vi "DateTimeMeasure.vi"(5 "EndTime":timestamp, 7 "StartTime":timestamp, 8 "error in":errorcluster, 11 "DateTimeMeasure":refnum<class "DateTimeMeasure.lvclass">) -> (0 "error out":errorcluster, 3 "Passed":bool)   [LabVIEW 2020]
uses:
  ProligentResultProcessor/Measure/DateTimeMeasure/DateTimeMeasure.lvclass
  C:/Projects/Result Processor/src/LabVIEWResultProcessor/ProligentResultProcessor/Measure/Measure/Measure.lvclass
  ProligentResultProcessor/Measure/DateTimeMeasureLimit/DateTimeMeasureLimit.lvclass
  C:/Projects/Result Processor/src/LabVIEWResultProcessor/ProligentResultProcessor/Measure/RangeMeasureLimit/RangeMeasureLimit.lvclass
  C:/Projects/Result Processor/src/LabVIEWResultProcessor/ProligentResultProcessor/Measure/MeasureLimit/MeasureLimit.lvclass
  ProligentResultProcessor/Measure/RangeMeasureLimit/ComparisonType.ctl
  ProligentResultProcessor/Measure/Measure/SetStartDate.vi
  ProligentResultProcessor/Measure/Measure/SetMeasureExecutionStatus.vi
  ProligentResultProcessor/Measure/DateTimeMeasure/SetValue.vi
  ProligentResultProcessor/Measure/Measure/SetComments.vi
  ProligentResultProcessor/Measure/Measure/SetMeasureId.vi
  ProligentResultProcessor/Measure/Measure/GetStartDate.vi
  ProligentResultProcessor/Measure/Measure/GetMeasureExecutionStatus.vi
  ProligentResultProcessor/Measure/DateTimeMeasure/GetValue.vi
  ProligentResultProcessor/Measure/Measure/GetComments.vi
  ProligentResultProcessor/Measure/Measure/GetMeasureId.vi
  ProligentResultProcessor/Measure/Measure/GetLimit.vi
  ProligentResultProcessor/Measure/DateTimeMeasureLimit/SetHigherBound.vi
  ProligentResultProcessor/Measure/DateTimeMeasureLimit/SetLowerBound.vi
  ProligentResultProcessor/Measure/RangeMeasureLimit/GetComparisonType.vi
  ProligentResultProcessor/Measure/DateTimeMeasureLimit/GetHigherBound.vi
  ProligentResultProcessor/Measure/DateTimeMeasureLimit/GetLowerBound.vi
  ProligentResultProcessor/Measure/MeasureLimit/GetLimitExpression.vi
  ProligentResultProcessor/Measure/MeasureLimit/GetCustomData.vi
  ProligentResultProcessor/Measure/MeasureLimit/MeasureLimit.lvclass
  ProligentResultProcessor/Model/CustomData/CustomData.lvclass
  ProligentResultProcessor/Measure/RangeMeasureLimit/RangeMeasureLimit.lvclass
  ProligentResultProcessor/Measure/Measure/Measure.lvclass
  C:/Projects/Result Processor/src/LabVIEWResultProcessor/ProligentResultProcessor/Measure/DateTimeMeasure/DateTimeMeasure.lvclass
  C:/Projects/Result Processor/src/LabVIEWResultProcessor/ProligentResultProcessor/Measure/DateTimeMeasureLimit/DateTimeMeasureLimit.lvclass
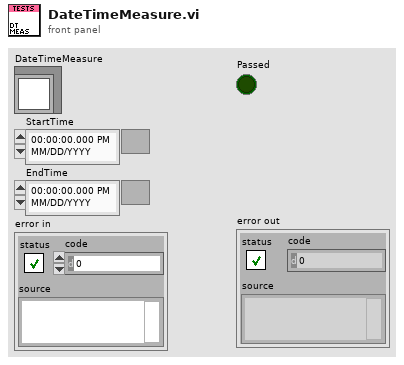
[diagram p1: front panel]
types:
  T1 = typedef "ProligentResultProcessor.lvlib/RangeMeasureLimit.lvclass/ComparisonType.ctl" = enum16{"LowerBound <= X <= HigherBound", "LowerBound < X <= HigherBound", "LowerBound <= X < HigherBound", "LowerBound < X < HigherBound", "LowerBound <= X", "LowerBound < X", "X <= HigherBound", "X < HigherBound", "X == HigherBound", "X != HigherBound", "X <= LowerBound OR HigherBound <= X", "X < LowerBound OR HigherBound <= X", "X <= LowerBound OR HigherBound < X", "X < LowerBound OR HigherBound < X"}
  T2 = enum16{"PASS", "FAIL", "NOT_COMPLETED", "ABORTED"}
  T3 = typedef "ProligentResultProcessor.lvlib/ExecutionStatus.lvclass/Value.ctl" = enum16{"PASS", "FAIL", "NOT_COMPLETED", "ABORTED"}
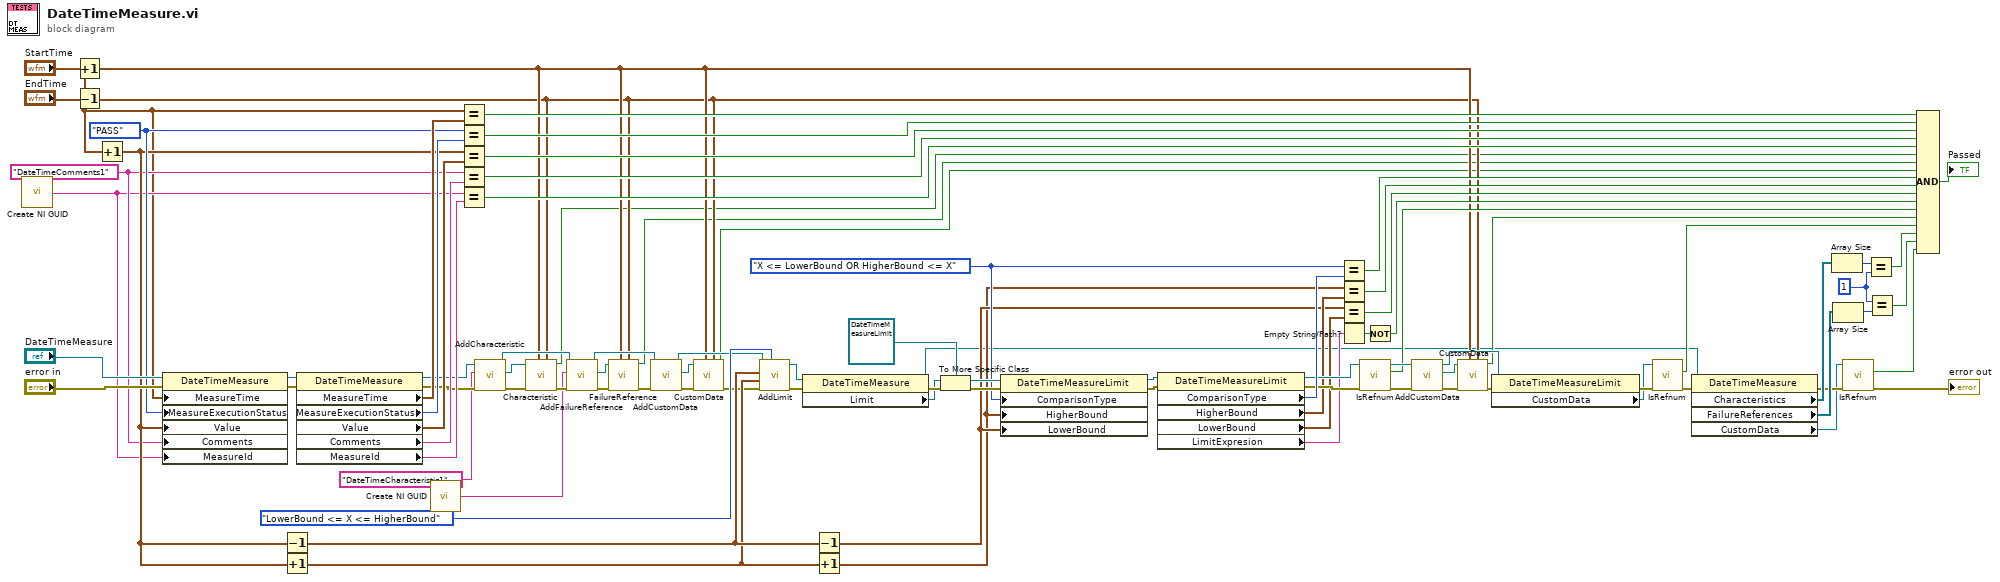
[diagram p0: block diagram]
diagram:
  w7 = 1
  w38 = "DateTimeComments1"
  w53 = ComparisonType."X <= LowerBound OR HigherBound <= X" ("ComparisonType")
  w79 = T2."PASS" ("ProcessRunStatus")
  n1 = call <vilib>:"Create NI GUID.vi"() -> ("NI GUID"=w35:string)
  n2 = Increment(x="StartTime") -> (x+1=w20:timestamp)
  n3 = Decrement(x="EndTime") -> (x-1=w19:timestamp)
  n4 = Increment(x=w20) -> (x+1=w47:timestamp)
  n5 = property class="DateTimeMeasure"(reference="DateTimeMeasure", error in="error in", "MeasureTime"=w20, "MeasureExecutionStatus"=w79, "Value"=w47, "Comments"=w38, "MeasureId"=w35) -> (reference out=w90:refnum<class "DateTimeMeasure.lvclass">, error out=w89:errorcluster)
  n6 = Decrement(x=w47) -> (x-1=w45:timestamp)
  n7 = Increment(x=w47) -> (x+1=w44:timestamp)
  n8 = property class="DateTimeMeasure"(reference=w90, error in=w89) -> (reference out=w22:refnum<class "DateTimeMeasure.lvclass">, error out=w24:errorcluster, "MeasureTime"=w88:timestamp, "MeasureExecutionStatus"=w87:T3, "Value"=w86:timestamp, "Comments"=w37:string, "MeasureId"=w36:string)
  n9 = call <vilib>:"Create NI GUID.vi"() -> ("NI GUID"=w17:string)
  n10 = Equal?(x=w20, y=w88) -> (x = y?=w85:bool)
  n11 = Equal?(x=w79, y=w87) -> (x = y?=w84:bool)
  n12 = Equal?(x=w47, y=w86) -> (x = y?=w83:bool)
  n13 = Equal?(x=w38, y=w37) -> (x = y?=w40:bool)
  n14 = Equal?(x=w35, y=w36) -> (x = y?=w39:bool)
  n15 = call "AddCharacteristic.vi"("error in (no error)"=w24, "FullName"="DateTimeCharacteristic1", "Measure in"=w22) -> ("error out"=w34:errorcluster, "Characteristic"=w33:refnum<class "Characteristic.lvclass">, "Measure out"=w31:refnum<class "DateTimeMeasure.lvclass">)  [unwired: 6 in]
  n16 = call "Characteristic.vi"("EndTime"=w19, "StartTime"=w20, "error in (no error)"=w34, "Characteristic in"=w33) -> ("error out"=w32:errorcluster, "Passed"=w16:bool)  [unwired: 6 in]
  n17 = call "AddFailureReference.vi"("error in (no error)"=w32, "Id"=w17, "Measure in"=w31) -> ("error out"=w26:errorcluster, "FailureReference"=w25:refnum<class "FailureReference.lvclass">, "Measure out"=w28:refnum<class "DateTimeMeasure.lvclass">)  [unwired: 6 in]
  n18 = call "FailureReference.vi"("EndTime"=w19, "StartTime"=w20, "error in"=w26, "Defect"=w25) -> ("error out"=w30:errorcluster, "Passed"=w15:bool)  [unwired: 6 in]
  n19 = call "AddCustomData.vi"("error in (no error)"=w30, "Measure in"=w28) -> ("error out"=w29:errorcluster, "CustomData"=w27:refnum<class "CustomData.lvclass">, "Measure out"=w21:refnum<class "DateTimeMeasure.lvclass">)  [unwired: 7 in]
  n20 = call "CustomData.vi"("EndTime"=w19, "StartTime"=w20, "error in"=w29, "CustomData"=w27) -> ("error out"=w23:errorcluster, "Passed"=w14:bool)  [unwired: 6 in]
  n21 = call "AddLimit.vi"("ComparisonType"=ComparisonType."LowerBound <= X <= HigherBound", "error in"=w23, "HigherBound"=w44, "LowerBound"=w45, "DateTimeMeasure in"=w21) -> ("error out"=w73:errorcluster, "DateTimeMeasure out"=w78:refnum<class "DateTimeMeasure.lvclass">)  [unwired: 4 in, 1 out]
  n22 = property class="DateTimeMeasure"(reference=w78, error in=w73) -> (reference out=w13:refnum<class "DateTimeMeasure.lvclass">, error out=w77:errorcluster, "Limit"=w74:refnum<class "MeasureLimit.lvclass">)
  n23 = Decrement(x=w45) -> (x-1=w43:timestamp)
  n24 = Increment(x=w44) -> (x+1=w42:timestamp)
  n25 = To More Specific Class(target class=refnum<class "DateTimeMeasureLimit.lvclass"> refnum ("ProligentResultProcessor:DateTimeMeasureLimit"), reference=w74, error in=w77) -> (specific class reference=w75:refnum<class "DateTimeMeasureLimit.lvclass">, error out=w76:errorcluster)
  n26 = property class="DateTimeMeasureLimit"(reference=w75, error in=w76, "ComparisonType"=w53, "HigherBound"=w42, "LowerBound"=w43) -> (reference out=w72:refnum<class "DateTimeMeasureLimit.lvclass">, error out=w71:errorcluster)
  n27 = property class="DateTimeMeasureLimit"(reference=w72, error in=w71) -> (reference out=w63:refnum<class "DateTimeMeasureLimit.lvclass">, error out=w68:errorcluster, "ComparisonType"=w70:T1, "HigherBound"=w52:timestamp, "LowerBound"=w51:timestamp, "LimitExpresion"=w54:string)
  n28 = Equal?(x=w53, y=w70) -> (x = y?=w50:bool)
  n29 = Equal?(x=w42, y=w52) -> (x = y?=w49:bool)
  n30 = Equal?(x=w43, y=w51) -> (x = y?=w48:bool)
  n31 = Empty String/Path?(string/path=w54) -> (empty?=w69:bool)
  n32 = call "IsRefnum.vi"("error in"=w68, "MeasureLimit in"=w63) -> ("error out"=w64:errorcluster, "IsRefnum"=w61:bool, "MeasureLimit out"=w62:refnum<class "DateTimeMeasureLimit.lvclass">)  [unwired: 7 in]
  n33 = Not(x=w69) -> (.not. x?=w41:bool)
  n34 = call "AddCustomData.vi"("error in"=w64, "MeasureLimit in"=w62) -> ("error out"=w59:errorcluster, "CustomData"=w57:refnum<class "CustomData.lvclass">, "MeasureLimit out"=w60:refnum<class "DateTimeMeasureLimit.lvclass">)  [unwired: 7 in]
  n35 = call "CustomData.vi"("EndTime"=w19, "StartTime"=w20, "error in"=w59, "CustomData"=w57) -> ("error out"=w58:errorcluster, "Passed"=w56:bool)  [unwired: 6 in]
  n36 = property class="DateTimeMeasureLimit"(reference=w60, error in=w58) -> (error out=w67:errorcluster, "CustomData"=w66:refnum<class "CustomData.lvclass">)  [unwired: 1 out]
  n37 = call "IsRefnum.vi"("error in"=w67, "CustomDataType in"=w66) -> ("error out"=w12:errorcluster, "IsRefnum"=w65:bool)  [unwired: 7 in, 1 out]
  n38 = property class="DateTimeMeasure"(reference=w13, error in=w12) -> (error out=w6:errorcluster, "Characteristics"=w11:refnum<class "Characteristic.lvclass">[], "FailureReferences"=w9:refnum<class "FailureReference.lvclass">[], "CustomData"=w4:refnum<class "CustomData.lvclass">)  [unwired: 1 out]
  n39 = Array Size(array=w11) -> (size(s)=w10:i32)
  n40 = Array Size(array=w9) -> (size(s)=w8:i32)
  n41 = call "IsRefnum.vi"("error in"=w6, "CustomDataType in"=w4) -> ("error out"=→"error out":errorcluster, "IsRefnum"=w1:bool)  [unwired: 7 in, 1 out]
  n42 = Equal?(x=w10, y=w7) -> (x = y?=w3:bool)
  n43 = Equal?(x=w7, y=w8) -> (x = y?=w2:bool)
  n44 = Compound Arithmetic op=AND(w85, w84, w83, w40, w39, w16, w15, w14, w50, w49, w48, w41, w61, w56, w65, w3, w2, w1) -> (→"Passed":bool)
